vi "网络通信.vi"() -> ()   [LabVIEW 2015]
panel:
  in  "目标IP":string caption="连接对象"
  in  "端口":u16
  in  "UDP连接":refnum<k16>
  in  "连接对象":u16(ring) items=["no connection"]
  in  "Multi Client ID":T1
  out "状态显示":string
  out "发送数据":i32
  in  "连接协议":enum16{"TCP Client", "TCP Server", "UDP"}(ring)
  in  "清空接收":bool
  in  "端口号":u16=1 caption="端 口 号:"
  in  "IP地址":string caption="IP  地 址"
  in  "连接":bool
  in  "发送":bool
  in  "数据接收":string
  in  "数据发送":string
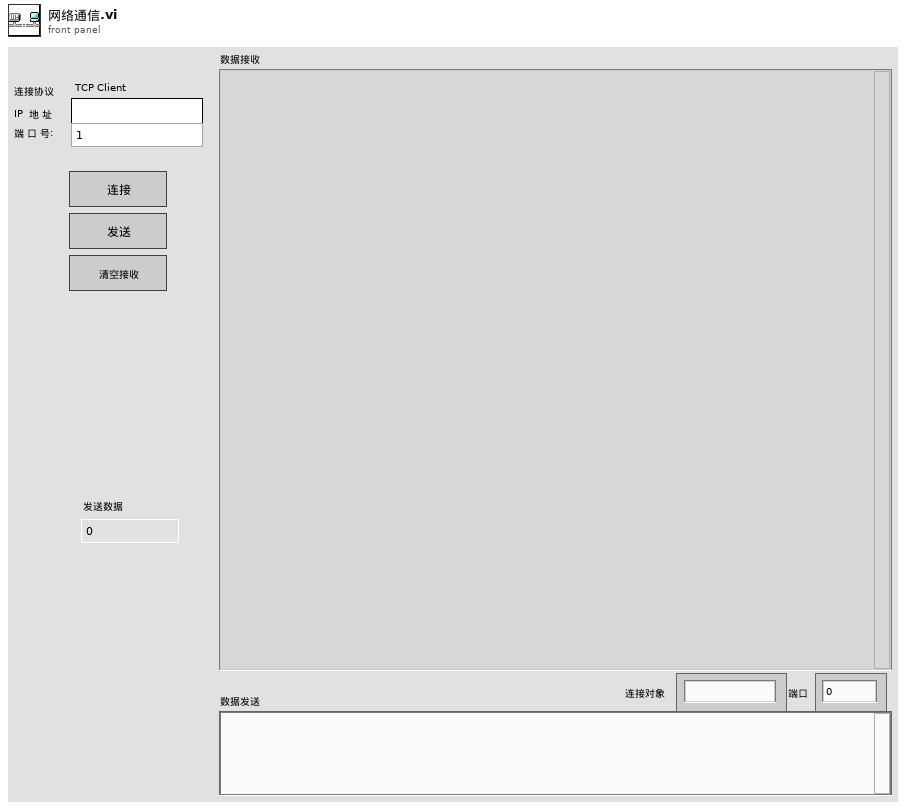
[diagram p1: front panel]
types:
  T1 = cluster{"Client":refnum<k5>[], "侦听器ID":refnum<k5>, "远程连接对象":cluster{"IP":string, "端口":u16}[]}
  T2 = enum16{"Initialization", "IDLE", "Connect", "S_Connect", "C_Read/Write", "C_Disconnect", "S_Read/Write", "S_Disconnect"}
  T3 = enum8{"Enabled", "Disabled", "Disabled and Grayed Out"}
  T4 = typedef "LVRectTypeDef.ctl" = cluster{"Left":i16, "Top":i16, "Right":i16, "Bottom":i16}
  T5 = typedef "LVPointTypeDef.ctl" = cluster{"Horizontal":i16, "Vertical":i16}
  T6 = cluster{"remote address":string, "remote port":u16}
  T7 = cluster{"remote address":string, "remote port":u16}[]
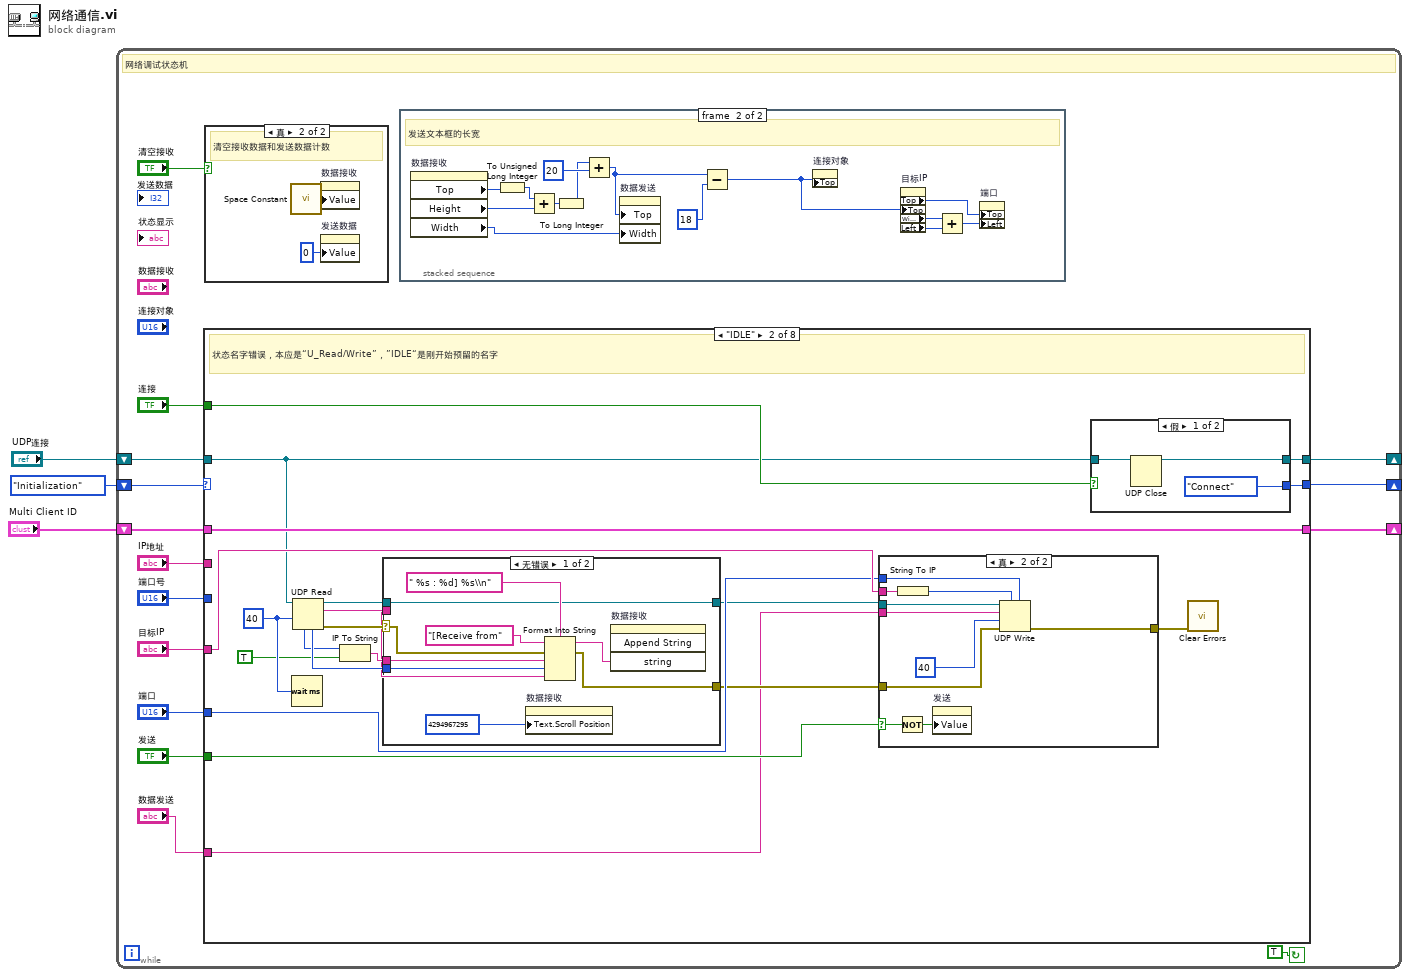
[diagram p0: block diagram]
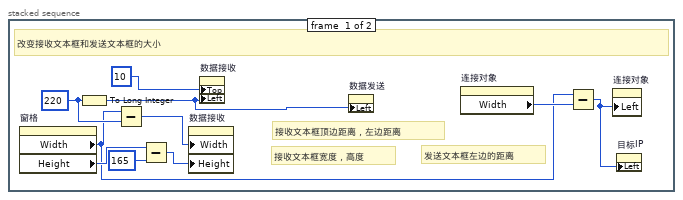
[diagram p2: hidden frame]
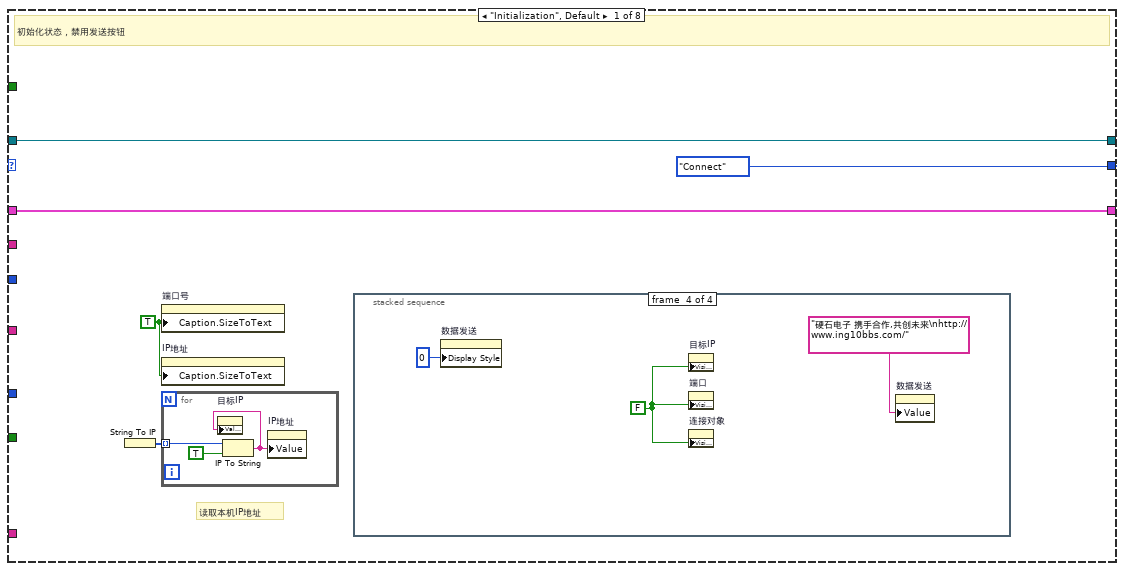
[diagram p4: hidden frame]
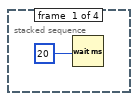
[diagram p5: hidden frame]
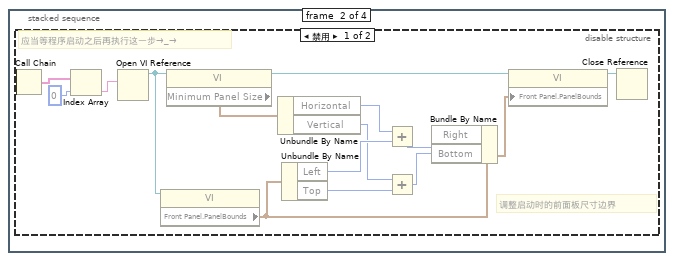
[diagram p6: hidden frame]
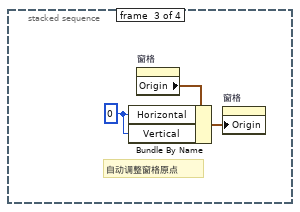
[diagram p8: hidden frame]
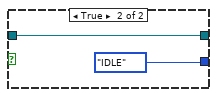
[diagram p9: hidden frame]
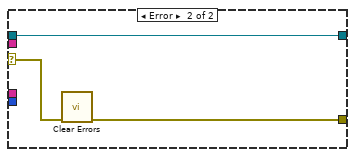
[diagram p11: hidden frame]
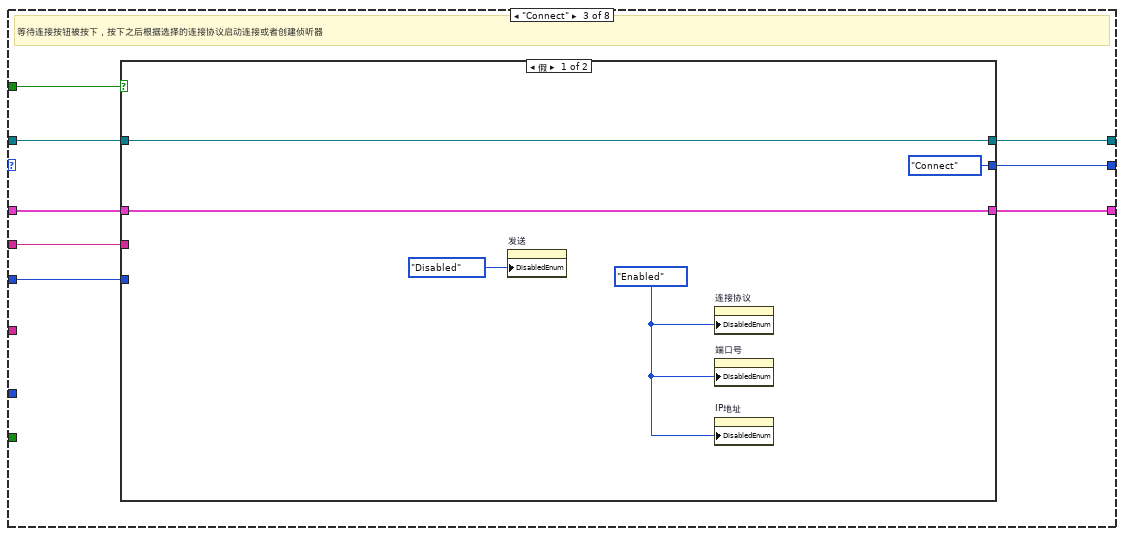
[diagram p12: hidden frame]
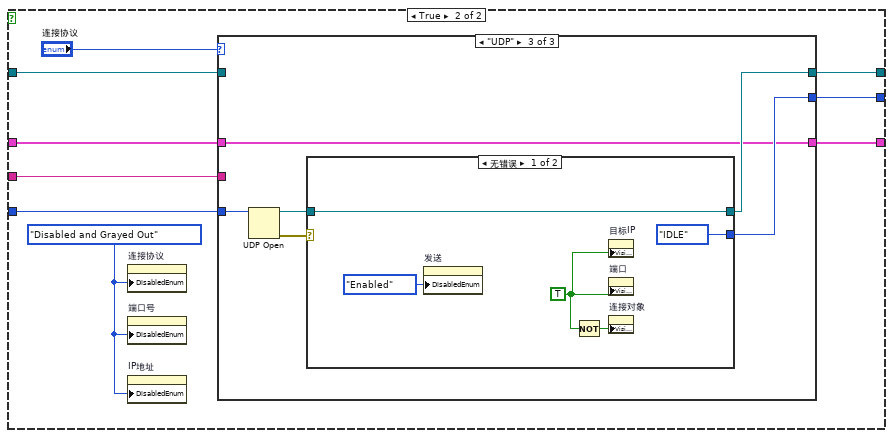
[diagram p13: hidden frame]
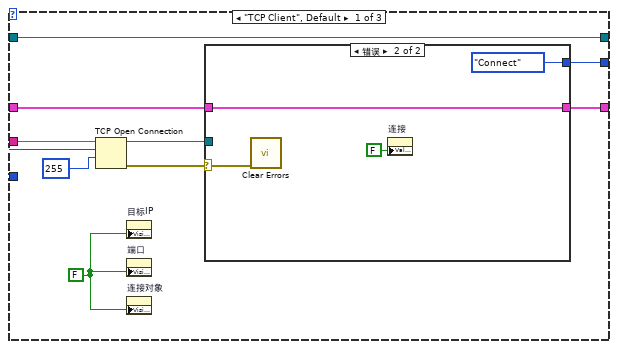
[diagram p14: hidden frame]
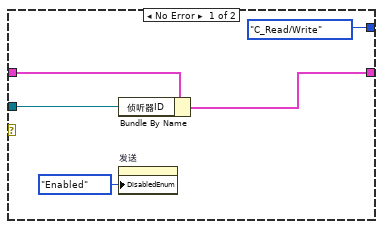
[diagram p15: hidden frame]
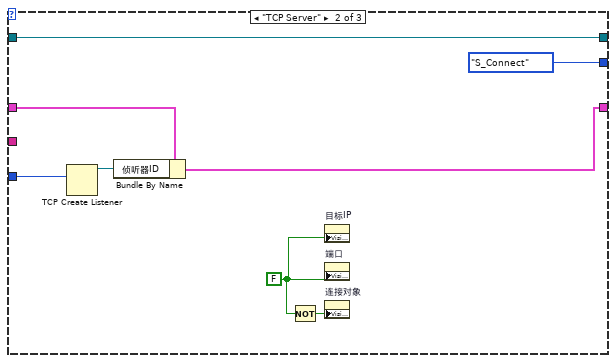
[diagram p16: hidden frame]
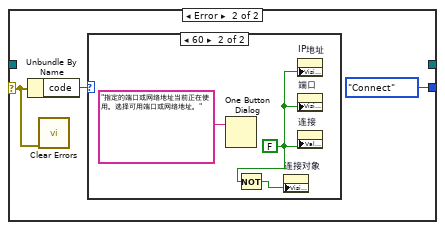
[diagram p17: hidden frame]
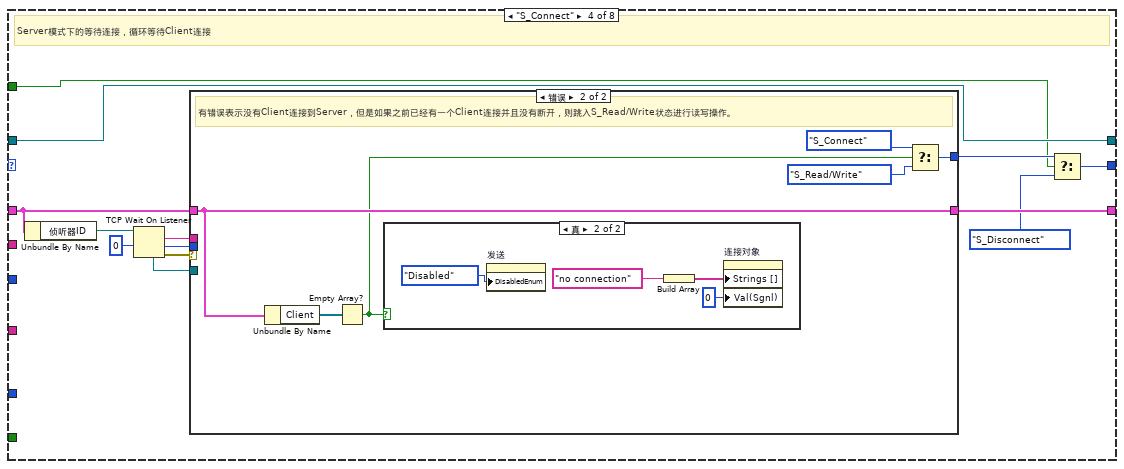
[diagram p19: hidden frame]
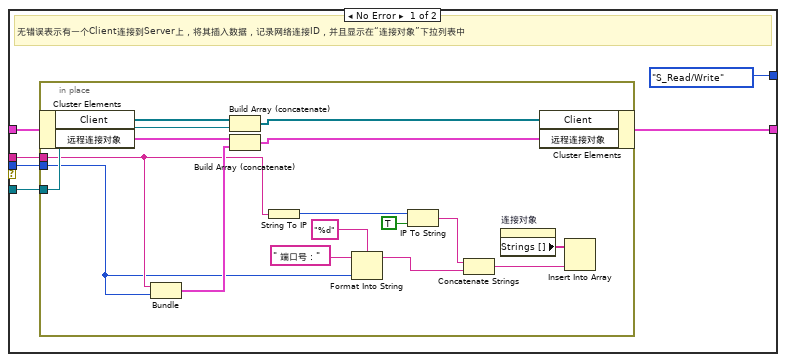
[diagram p20: hidden frame]
diagram:
  n1 = while "While循环" {
    shift-right: [w14] -> _
    shift-left: "Multi Client ID" -> [w15]
    shift-right: [w12] -> _
    shift-left: T2."Initialization" -> [w13]
    shift-right: [w9] -> _
    shift-left: "UDP连接" -> [w10]
    stop <- TRUE continue-if-true
    # "网络调试状态机"
    n2 = case "条件结构" shown="\"IDLE\"" w13 {
      tunnel: "IP地址" -> [_ _ w131 _ _ _ _ _]
      tunnel: "端口号" -> [_ _ w130 _ _ _ _ _]
      tunnel: w15 -> [w49 w94 w129 w198 w242 w267 w281 w344]
      tunnel: [w49 w94 w128 w197 w242 w267 w280 w344] -> w14
      tunnel: [T2."Connect" w93 w127 w192 w249 T2."Connect" w279 T2."Connect"] -> w12
      tunnel: w10 -> [w47 w76 w126 w191 w239 w266 w276 w338]
      tunnel: [w47 w75 w125 w191 w239 w266 w276 w338] -> w9
      tunnel: "目标IP" -> [_ w89 _ _ _ _ _ _]
      tunnel: "端口" -> [_ w88 _ _ _ _ _ _]
      tunnel: "发送" -> [_ w79 _ _ w238 _ w274 _]
      tunnel: "连接" -> [_ w77 w124 w190 w237 _ w273 _]
      tunnel: "数据发送" -> [_ w78 _ _ w236 _ w272 _]
      frame "Initialization", Default {
        w45 = TRUE
        # "读取本机IP地址"
        # "初始化状态，禁用发送按钮"
        n3 = String To IP() -> (0:w46:u32[])  [unwired: 1 out]
        n4 = property on="端口号" class="DigNum (严格)"("Caption.SizeToText"=w45) -> ()  [unwired: 2 in, 2 out]
        n5 = property on="IP地址" class="Str"("Caption.SizeToText"=w45) -> ()  [unwired: 2 in, 2 out]
        n6 = for {
          tunnel: w46 -> [w73] mode=indexing
          n7 = IP To String(1:TRUE ("dot notation? (F)"), 2:w73) -> (0:w72:string)
          n8 = property on="目标IP" class="Str"("Value"=w72) -> ()  [unwired: 2 in, 2 out]
          n9 = property on="IP地址" class="Str"("Value"=w72) -> ()  [unwired: 2 in, 2 out]
        }
        n10 = stacked-sequence {
          frame #0 {
            n11 = Wait (ms)(milliseconds to wait=u32 20) -> ()  [unwired: 1 out]
          }
          frame #1 {
            n12 = disable-structure shown="禁用" {
              frame Disabled {
                # "调整启动时的前面板尺寸边界"
                # "应当等程序启动之后再执行这一步→_→"
                n13 = Call Chain ("调用链")() -> (call chain=w53:string[])
                n14 = Index Array(array=w53, index=0) -> (element=w51:string)
                n15 = Open VI Reference(vi path=w51) -> (vi reference=w63:refnum<vi>)  [unwired: 1 in, 5 out]
                n16 = property class="VI"(reference=w63) -> ("Front Panel.PanelBounds"=w60:T4)  [unwired: 1 in, 2 out]
                n17 = property class="VI"(reference=w63) -> (reference out=w64:refnum<vi>, "Minimum Panel Size"=w54:T5)  [unwired: 1 in, 1 out]
                n18 = Unbundle By Name(w54) -> ("Horizontal"=w61:i16, "Vertical"=w58:i16)
                n19 = Unbundle By Name(w60) -> ("Left"=w62:i16, "Top"=w57:i16)
                n20 = Add(x=w61, y=w62) -> (x+y=w59:i16)
                n21 = Add(x=w58, y=w57) -> (x+y=w56:i16)
                n22 = Bundle By Name(cluster=w60, "Right"=w59, "Bottom"=w56) -> (w55:T4)
                n23 = property class="VI"(reference=w64, "Front Panel.PanelBounds"=w55) -> (reference out=w65:refnum<vi>)  [unwired: 1 in, 1 out]
                n24 = Close Reference(reference=w65) -> ()  [unwired: 1 in, 1 out]
              }
              frame Enabled {
              }
            }
          }
          frame #2 {
            w68 = i16 0
            # "自动调整窗格原点"
            n25 = property on="窗格" class="Pane"() -> ("Origin"=w67:T5)  [unwired: 2 in, 2 out]
            n26 = Bundle By Name(cluster=w67, "Horizontal"=w68, "Vertical"=w68) -> (w66:T5)
            n27 = property on="窗格" class="Pane"("Origin"=w66) -> ()  [unwired: 2 in, 2 out]
          }
          frame #3 {
            w69 = FALSE
            n28 = property on="数据发送" class="Str"("Display Style"=u32 0) -> ()  [unwired: 2 in, 2 out]
            n29 = property on="目标IP" class="Str"("Visible"=w69) -> ()  [unwired: 2 in, 2 out]
            n30 = property on="端口" class="DigNum (严格)"("Visible"=w69) -> ()  [unwired: 2 in, 2 out]
            n31 = property on="连接对象" class="Ring (严格)"("Visible"=w69) -> ()  [unwired: 2 in, 2 out]
            n32 = property on="数据发送" class="Str"("Value"="硬石电子 携手合作,共创未来\nhttp://www.ing10bbs.com/") -> ()  [unwired: 2 in, 2 out]
          }
        }
      }
      frame "IDLE" {
        w87 = 40
        # "状态名字错误，本应是“U_Read/Write”，”IDLE“是刚开始预留的名字"
        n33 = Wait (ms)(milliseconds to wait=w87) -> ()  [unwired: 1 out]
        n34 = UDP Read(connection ID=w76, timeout ms (25000)=w87) -> (data out=w91:string, error out=w92:errorcluster, 3:w86:refnum<k16>, 4:w90:u16, 6:w84:u32)  [unwired: 2 in]
        n35 = IP To String(1:TRUE, 2:w84) -> (0:w82:string)
        n36 = case shown="无错误" w92 {
          selector: w92 -> [w116 w123]
          tunnel: w91 -> [w118 _]
          tunnel: w90 -> [w119 _]
          tunnel: [w115 w122] -> w85
          tunnel: w86 -> [w115 w122]
          tunnel: w82 -> [w113 _]
          tunnel: [w112 w121] -> w81
          frame No Error {
            n37 = property on="数据接收" class="Str"("Text.Scroll Position"=u32 4294967295) -> ()  [unwired: 2 in, 2 out]
            n38 = Format Into String(format string=" %s : %d] %s\\n", initial string="[Receive from", error in=w116, w113, w119, w118) -> (resulting string=w117:string, error out=w112:errorcluster)
            n39 = invoke on="数据接收" class="Str" method="Append String"("string"=w117) -> ()  [unwired: 3 in, 4 out]
          }
          frame Error {
            n40 = call <vilib>:"Clear Errors.vi"("error in (no error)"=w123) -> ("error out"=w121:errorcluster)  [unwired: 5 in, 1 out]
          }
        }
        n41 = case shown="真" w79 {
          selector: w79 -> [_ w105]
          tunnel: w89 -> [_ w110]
          tunnel: w88 -> [_ w108]
          tunnel: w85 -> [_ w107]
          tunnel: w81 -> [w100 w103]
          tunnel: [w100 w102] -> w80
          tunnel: w78 -> [_ w101]
          frame False {
          }
          frame True {
            n42 = Not(x=w105) -> (.not. x?=w104:bool)
            n43 = String To IP(1:w110) -> (0:w109:u32)
            n44 = property on="发送" class="Bool (严格)"("Value"=w104) -> ()  [unwired: 2 in, 2 out]
            n45 = UDP Write(address=w109, port or service name=w108, connection ID=w107, data in=w101, 8:w103, 9:40) -> (error out=w102:errorcluster)  [unwired: 1 out]
          }
        }
        n46 = case shown="假" w77 {
          tunnel: [T2."Connect" T2."IDLE"] -> w93
          tunnel: w76 -> [w96 w98]
          tunnel: [w95 w98] -> w75
          frame False {
            n47 = UDP Close(connection ID=w96) -> (connection ID out=w95:refnum<k16>)  [unwired: 1 in, 1 out]
          }
          frame True {
          }
        }
        n48 = call <vilib>:"Clear Errors.vi"("error in (no error)"=w80) -> ()  [unwired: 5 in, 2 out]
      }
      frame "Connect" {
        # "等待连接按钮被按下，按下之后根据选择的连接协议启动连接或者创建侦听器"
        n49 = case shown="假" w124 {
          tunnel: w131 -> [_ w144]
          tunnel: w130 -> [_ w143]
          tunnel: w129 -> [w136 w142]
          tunnel: [w136 w141] -> w128
          tunnel: [T2."Connect" w140] -> w127
          tunnel: w126 -> [w133 w139]
          tunnel: [w133 w138] -> w125
          frame False {
            w132 = T3."Enabled"
            n50 = property on="发送" class="Bool (严格)"("DisabledEnum"=T3."Disabled") -> ()  [unwired: 2 in, 2 out]
            n51 = property on="连接协议" class="Enum (严格)"("DisabledEnum"=w132) -> ()  [unwired: 2 in, 2 out]
            n52 = property on="端口号" class="DigNum (严格)"("DisabledEnum"=w132) -> ()  [unwired: 2 in, 2 out]
            n53 = property on="IP地址" class="Str"("DisabledEnum"=w132) -> ()  [unwired: 2 in, 2 out]
          }
          frame True {
            w137 = T3."Disabled and Grayed Out"
            n54 = property on="连接协议" class="Enum (严格)"("DisabledEnum"=w137) -> ()  [unwired: 2 in, 2 out]
            n55 = property on="端口号" class="DigNum (严格)"("DisabledEnum"=w137) -> ()  [unwired: 2 in, 2 out]
            n56 = property on="IP地址" class="Str"("DisabledEnum"=w137) -> ()  [unwired: 2 in, 2 out]
            n57 = case shown="\"UDP\"" "连接协议" {
              tunnel: w144 -> [w155 _ _]
              tunnel: w143 -> [w154 w172 w178]
              tunnel: w142 -> [w151 w171 w173]
              tunnel: [w149 w169 w173] -> w141
              tunnel: [w148 T2."S_Connect" w176] -> w140
              tunnel: w139 -> [w147 w167 _]
              tunnel: [w147 w167 w174] -> w138
              frame "TCP Client", Default {
                w146 = FALSE
                n58 = TCP Open Connection(address=w155, remote port or service name=w154, timeout ms (60000)=255) -> (connection ID=w150:refnum<k5>, error out=w152:errorcluster)  [unwired: 2 in]
                n59 = property on="目标IP" class="Str"("Visible"=w146) -> ()  [unwired: 2 in, 2 out]
                n60 = property on="端口" class="DigNum (严格)"("Visible"=w146) -> ()  [unwired: 2 in, 2 out]
                n61 = property on="连接对象" class="Ring (严格)"("Visible"=w146) -> ()  [unwired: 2 in, 2 out]
                n62 = case shown="错误" w152 {
                  selector: w152 -> [_ w164]
                  tunnel: [w158 w163] -> w149
                  tunnel: [T2."C_Read/Write" T2."Connect"] -> w148
                  tunnel: w151 -> [w160 w163]
                  tunnel: w150 -> [w159 _]
                  frame No Error {
                    n63 = Bundle By Name(cluster=w160, "侦听器ID"=w159) -> (w158:T1)
                    n64 = property on="发送" class="Bool (严格)"("DisabledEnum"=T3."Enabled") -> ()  [unwired: 2 in, 2 out]
                  }
                  frame Error {
                    n65 = call <vilib>:"Clear Errors.vi"("error in (no error)"=w164) -> ()  [unwired: 5 in, 2 out]
                    n66 = property on="连接" class="Bool (严格)"("Value"=FALSE) -> ()  [unwired: 2 in, 2 out]
                  }
                }
              }
              frame "TCP Server" {
                w166 = FALSE
                n67 = TCP Create Listener(10:w172) -> (3:w170:refnum<k5>)  [unwired: 4 in, 2 out]
                n68 = Bundle By Name(cluster=w171, "侦听器ID"=w170) -> (w169:T1)
                n69 = Not(x=w166) -> (.not. x?=w165:bool)
                n70 = property on="目标IP" class="Str"("Visible"=w166) -> ()  [unwired: 2 in, 2 out]
                n71 = property on="端口" class="DigNum (严格)"("Visible"=w166) -> ()  [unwired: 2 in, 2 out]
                n72 = property on="连接对象" class="Ring (严格)"("Visible"=w165) -> ()  [unwired: 2 in, 2 out]
              }
              frame "UDP" {
                n73 = UDP Open(11:w178) -> (port=w175:refnum<k16>, 0:w177:errorcluster)  [unwired: 4 in, 1 out]
                n74 = case shown="无错误" w177 {
                  selector: w177 -> [_ w184]
                  tunnel: [T2."IDLE" T2."Connect"] -> w176
                  tunnel: w175 -> [w182 _]
                  tunnel: [w182 _] -> w174
                  frame No Error {
                    w180 = TRUE
                    n75 = property on="发送" class="Bool (严格)"("DisabledEnum"=T3."Enabled") -> ()  [unwired: 2 in, 2 out]
                    n76 = Not(x=w180) -> (.not. x?=w179:bool)
                    n77 = property on="目标IP" class="Str"("Visible"=w180) -> ()  [unwired: 2 in, 2 out]
                    n78 = property on="端口" class="DigNum (严格)"("Visible"=w180) -> ()  [unwired: 2 in, 2 out]
                    n79 = property on="连接对象" class="Ring (严格)"("Visible"=w179) -> ()  [unwired: 2 in, 2 out]
                  }
                  frame Error {
                    n80 = Unbundle By Name(w184) -> ("code"=w185:i32)
                    n81 = call <vilib>:"Clear Errors.vi"("error in (no error)"=w184) -> ()  [unwired: 5 in, 2 out]
                    n82 = case shown="60" w185 {
                      frame 0, Default {
                      }
                      frame 60 {
                        w187 = FALSE
                        n83 = One Button Dialog(message="指定的端口或网络地址当前正在使用。选择可用端口或网络地址。") -> ()  [unwired: 1 in, 1 out]
                        n84 = Not(x=w187) -> (.not. x?=w188:bool)
                        n85 = property on="连接对象" class="Ring (严格)"("Visible"=w188) -> ()  [unwired: 2 in, 2 out]
                        n86 = property on="IP地址" class="Str"("Visible"=w187) -> ()  [unwired: 2 in, 2 out]
                        n87 = property on="端口" class="DigNum (严格)"("Visible"=w187) -> ()  [unwired: 2 in, 2 out]
                        n88 = property on="连接" class="Bool (严格)"("Value"=w187) -> ()  [unwired: 2 in, 2 out]
                      }
                    }
                  }
                }
              }
            }
          }
        }
      }
      frame "S_Connect" {
        # "Server模式下的等待连接，循环等待Client连接"
        n89 = Unbundle By Name(w198) -> ("侦听器ID"=w201:refnum<k5>)
        n90 = TCP Wait On Listener(9:0 ("超时时间(ms)"), 11:w201) -> (0:w202:errorcluster, 1:w196:u16, 2:w195:string, 4:w199:refnum<k5>)  [unwired: 2 in, 1 out]
        n91 = case "条件结构" shown="错误" w202 {
          tunnel: w199 -> [w208 _]
          tunnel: w198 -> [w204 w228]
          tunnel: [w206 w228] -> w197
          tunnel: [T2."S_Read/Write" w229] -> w193
          tunnel: w196 -> [w205 _]
          tunnel: w195 -> [w203 _]
          frame No Error {
            # "无错误表示有一个Client连接到Server上，将其插入数据，记录网络连接ID，并且显示在“连接对象”下拉列表中"
            n92 = in-place {
              in-place-border: w208 -> [w222]
              in-place-border: w205 -> [w211]
              in-place-border: w203 -> [w212]
              n93 = in-place-cluster #1(w204) -> ("Client"=w224:refnum<k5>[], "远程连接对象"=w215:cluster{"IP":string, "端口":u16}[])
              n94 = Bundle("remote address"=w212, "remote port"=w211) -> (w213:T6)  [unwired: 1 in]
              n95 = Build Array (concatenate)(w224, w222) -> (w223:refnum<k5>[])
              n96 = Build Array (concatenate)(w215, w213) -> (w214:T7)
              n97 = String To IP(1:w212) -> (0:w216:u32)
              n98 = Format Into String(format string="%d", initial string=" 端口号：", w211) -> (resulting string=w221:string)  [unwired: 1 in, 1 out]
              n99 = IP To String(1:TRUE, 2:w216) -> (0:w218:string)
              n100 = Concatenate Strings(w218, w221) -> (w210:string)
              n101 = property on="连接对象" class="Ring (严格)"() -> ("Strings []"=w209:string[])  [unwired: 2 in, 2 out]
              n102 = in-place-cluster #1("Client"=w223, "远程连接对象"=w214) -> (w206:T1)
              n103 = Insert Into Array(array=w209, new element=w210) -> ()  [unwired: 1 in, 1 out]
            }
          }
          frame Error {
            # "有错误表示没有Client连接到Server，但是如果之前已经有一个Client连接并且没有断开，则跳入S_Read/Write状态进行读写操作。"
            n104 = Unbundle By Name(w228) -> ("Client"=w230:refnum<k5>[])
            n105 = Empty Array?(array=w230) -> (empty?=w225:bool)
            n106 = case shown="真" w225 {
              frame False {
                n107 = property on="发送" class="Bool (严格)"("DisabledEnum"=T3."Enabled") -> ()  [unwired: 2 in, 2 out]
              }
              frame True {
                n108 = property on="发送" class="Bool (严格)"("DisabledEnum"=T3."Disabled") -> ()  [unwired: 2 in, 2 out]
                n109 = Build Array("no connection") -> (w234:string[])
                n110 = property on="连接对象" class="Ring (严格)"("Strings []"=w234, "Val(Sgnl)"=u16 0) -> ()  [unwired: 2 in, 2 out]
              }
            }
            n111 = Select(t=T2."S_Connect", s=w225, f=T2."S_Read/Write") -> (s? t:f=w229:T2)
          }
        }
        n112 = Select(t=w193, s=w190, f=T2."S_Disconnect") -> (s? t:f=w192:T2)
      }
      frame "C_Read/Write" {
        # "Client 模式下的读写状态"
        n113 = Unbundle By Name(w242) -> ("侦听器ID"=w243:refnum<k5>)
        n114 = TCP Read(connection ID=w243, bytes to read=1, 9:0) -> (connection ID out=w245:refnum<k5>, data out=w246:string, error out=w247:errorcluster)  [unwired: 2 in]
        n115 = case shown="无错误" w247 {
          selector: w247 -> [_ w260]
          tunnel: w246 -> [w259 _]
          tunnel: w245 -> [_ w261]
          frame No Error {
            # "无错误，能读取到数据"
            n116 = invoke on="数据接收" class="Str" method="Append String"("string"=w259) -> ()  [unwired: 3 in, 4 out]
            n117 = property on="数据接收" class="Str"("Text.Scroll Position"=u32 4294967295) -> ()  [unwired: 2 in, 2 out]
          }
          frame Error {
            # "有错误，但超时可以忽略"
            n118 = Unbundle By Name(w260) -> ("code"=w262:i32)
            n119 = case shown="66" w262 {
              tunnel: w261 -> [_ _ _]
              tunnel: w260 -> [w263 _ w265]
              frame 0, Default {
                # "其他错误"
                n120 = call <vilib>:"Clear Errors.vi"("error in (no error)"=w263) -> ()  [unwired: 5 in, 2 out]
              }
              frame 56 {
                # "连接超时，表示无错误"
              }
              frame 66 {
                # "断开连接"
                n121 = call <vilib>:"Clear Errors.vi"("error in (no error)"=w265) -> ()  [unwired: 5 in, 2 out]
                n122 = property on="连接" class="Bool (严格)"("Value"=FALSE) -> ()  [unwired: 2 in, 2 out]
              }
            }
          }
        }
        n123 = case shown="真" w238 {
          selector: w238 -> [_ w255]
          tunnel: w243 -> [_ w257]
          tunnel: w236 -> [_ w250]
          frame False {
          }
          frame True {
            n124 = Not(x=w255) -> (.not. x?=w254:bool)
            n125 = property on="发送" class="Bool (严格)"("Value"=w254) -> ()  [unwired: 2 in, 2 out]
            n126 = TCP Write(connection ID=w257, data in=w250) -> (bytes written=w252:i32, error out=w256:errorcluster)  [unwired: 2 in, 1 out]
            n127 = call <vilib>:"Clear Errors.vi"("error in (no error)"=w256) -> ()  [unwired: 5 in, 2 out]
            n128 = property on="发送数据" class="DigNum (严格)"() -> ("Value"=w253:i32)  [unwired: 2 in, 2 out]
            n129 = Add(x=w253, y=w252) -> (x+y=w251:i32)
            n130 = property on="发送数据" class="DigNum (严格)"("Value"=w251) -> ()  [unwired: 2 in, 2 out]
          }
        }
        n131 = Select(t=T2."C_Read/Write", s=w237, f=T2."C_Disconnect") -> (s? t:f=w249:T2)
      }
      frame "C_Disconnect" {
        # "Client 模式下的断开连接状态，进入这个状态只有两种可能，一种是Server 断开连接，另一种是Client主动断开连接（按下断开连接按钮）"
        n132 = Unbundle By Name(w267) -> ("侦听器ID"=w271:refnum<k5>)
        n133 = TCP Close Connection(connection ID=w271) -> (error out=w270:errorcluster)  [unwired: 2 in, 1 out]
        n134 = call <vilib>:"Clear Errors.vi"("error in (no error)"=w270) -> ()  [unwired: 5 in, 2 out]
        n135 = property on="发送" class="Bool (严格)"("DisabledEnum"=T3."Disabled") -> ()  [unwired: 2 in, 2 out]
      }
      frame "S_Read/Write" {
        # "状态机实现Server模式的读写状态，轮询各个Client的数据，有数据则显示，无数据则超时无响应，如果断开连接则删除网络连接句柄ID。写数据到Client的时候，则根据下拉列表所选择的Client作为连接对象。"
        n136 = in-place {
          in-place-border: [w292] -> w275
          n137 = in-place-cluster #2(w281) -> ("Client"=w292:refnum<k5>[], "远程连接对象"=w294:cluster{"IP":string, "端口":u16}[])
          n138 = for {
            tunnel: [w311] -> w296 mode=indexing if=w299
            tunnel: w292 -> [w310] mode=indexing
            tunnel: w294 -> [w298] mode=indexing
            tunnel: [w308] -> w295 mode=indexing if=w299
            tunnel: [w297] -> w293 mode=indexing if=w299
            n139 = TCP Read(connection ID=w310, bytes to read=1, 9:0) -> (connection ID out=w312:refnum<k5>, data out=w313:string, error out=w314:errorcluster)  [unwired: 2 in]
            n140 = case "条件结构" shown="无错误" w314 {
              selector: w314 -> [_ w324]
              tunnel: w313 -> [w320 _]
              tunnel: w312 -> [w319 w326]
              tunnel: [w319 w325] -> w311
              tunnel: [TRUE w323] -> w299
              tunnel: [w318 w322] -> w308
              tunnel: w298 -> [w318 w321]
              frame No Error {
                # "无错误，能读取到数据"
                # "Client有发送数据，追加到接受文本框字符串结尾"
                n141 = invoke on="数据接收" class="Str" method="Append String"("string"=w320) -> ()  [unwired: 3 in, 4 out]
                n142 = property on="数据接收" class="Str"("Text.Scroll Position"=u32 4294967295) -> ()  [unwired: 2 in, 2 out]
              }
              frame Error {
                # "有错误，但超时可以忽略"
                n143 = Unbundle By Name(w324) -> ("code"=w327:i32)
                n144 = case "条件结构" shown="66" w327 {
                  tunnel: w326 -> [_ w332 w337]
                  tunnel: [_ w332 _] -> w325
                  tunnel: w324 -> [w329 _ w334]
                  tunnel: [FALSE TRUE FALSE] -> w323
                  tunnel: [_ w331 _] -> w322
                  tunnel: w321 -> [_ w331 _]
                  frame 0, Default {
                    # "其他错误"
                    n145 = call <vilib>:"Clear Errors.vi"("error in (no error)"=w329) -> ()  [unwired: 5 in, 2 out]
                  }
                  frame 56 {
                    # "连接超时，表示无错误"
                    # "超时错误，当没有断开连接，只是Client没有发送数据而已"
                  }
                  frame 66 {
                    # "断开连接"
                    # "Client 断开连接，关闭连接，注销句柄ID"
                    n146 = TCP Close Connection(connection ID=w337, error in (no error)=w334) -> (error out=w333:errorcluster)  [unwired: 1 in, 1 out]
                    n147 = call <vilib>:"Clear Errors.vi"("error in (no error)"=w333) -> ()  [unwired: 5 in, 2 out]
                    n148 = property on="连接对象" class="Ring (严格)"("Val(Sgnl)"=0) -> ()  [unwired: 2 in, 2 out]
                  }
                }
              }
            }
            n149 = Unbundle(w308) -> ("IP"=w307:string, "端口"=w300:u16)
            n150 = String To IP(1:w307) -> (0:w306:u32)
            n151 = Format Into String(format string="%d", initial string=" 端口号：", w300) -> (resulting string=w304:string)  [unwired: 1 in, 1 out]
            n152 = IP To String(1:TRUE, 2:w306) -> (0:w301:string)
            n153 = Concatenate Strings(w301, w304) -> (w297:string)
          }
          n154 = in-place-cluster #2("Client"=w296, "远程连接对象"=w295) -> (w280:T1)
          n155 = property on="连接对象" class="Ring (严格)"("Strings []"=w293) -> ()  [unwired: 2 in, 2 out]
        }
        n156 = case "条件结构" shown="真" w274 {
          selector: w274 -> [_ w290]
          tunnel: w275 -> [_ w289]
          tunnel: w272 -> [_ w282]
          frame False {
          }
          frame True {
            # "发送数据，根据下拉列表的内容来选择发送数据的对象"
            n157 = property on="连接对象" class="Ring (严格)"() -> ("Value"=w286:u16)  [unwired: 2 in, 2 out]
            n158 = Not(x=w290) -> (.not. x?=w291:bool)
            n159 = property on="发送" class="Bool (严格)"("Value"=w291) -> ()  [unwired: 2 in, 2 out]
            n160 = Index Array(array=w289, index=w286) -> (element=w288:refnum<k5>)
            n161 = TCP Write(connection ID=w288, data in=w282) -> (bytes written=w284:i32, error out=w287:errorcluster)  [unwired: 2 in, 1 out]
            n162 = property on="发送数据" class="DigNum (严格)"() -> ("Value"=w285:i32)  [unwired: 2 in, 2 out]
            n163 = call <vilib>:"Clear Errors.vi"("error in (no error)"=w287) -> ()  [unwired: 5 in, 2 out]
            n164 = Add(x=w285, y=w284) -> (x+y=w283:i32)
            n165 = property on="发送数据" class="DigNum (严格)"("Value"=w283) -> ()  [unwired: 2 in, 2 out]
          }
        }
        n166 = Select(t=T2."S_Connect", s=w273, f=T2."S_Disconnect") -> (s? t:f=w279:T2)
      }
      frame "S_Disconnect" {
        w340 = u16 0
        # "Server状态下断开连接，关闭所有连接句柄，注销网络连接ID"
        n167 = Unbundle By Name(w344) -> ("Client"=w348:refnum<k5>[], "侦听器ID"=w349:refnum<k5>)
        n168 = TCP Close Connection(connection ID=w349) -> (error out=w347:errorcluster)  [unwired: 2 in, 1 out]
        n169 = for {
          tunnel: w348 -> [w352] mode=indexing
          shift-right: [w350] -> w346
          shift-left: w347 -> [w351]
          n170 = TCP Close Connection(connection ID=w352, error in (no error)=w351) -> (error out=w350:errorcluster)  [unwired: 1 in, 1 out]
        }
        n171 = property on="发送" class="Bool (严格)"("DisabledEnum"=T3."Disabled") -> ()  [unwired: 2 in, 2 out]
        n172 = property on="连接对象" class="Ring (严格)"("Val(Sgnl)"=w340) -> ()  [unwired: 2 in, 2 out]
        n173 = Bundle("no connection", w340) -> (w342:cluster{string, u16})  [unwired: 1 in]
        n174 = call <vilib>:"Clear Errors.vi"("error in (no error)"=w346) -> ()  [unwired: 5 in, 2 out]
        n175 = Build Array(w342) -> (w341:cluster{string, u16}[])
        n176 = property on="连接对象" class="Ring (严格)"("StringsAndValues[]"=w341) -> ()  [unwired: 2 in, 2 out]
      }
    }
    n177 = case "条件结构" shown="真" "清空接收" {
      frame False {
      }
      frame True {
        # "清空接收数据和发送数据计数"
        n178 = call <vilib>:"Space Constant.vi"() -> ("String"=w44:string)
        n179 = property on="数据接收" class="Str"("Value"=w44) -> ()  [unwired: 2 in, 2 out]
        n180 = property on="发送数据" class="DigNum (严格)"("Value"=0) -> ()  [unwired: 2 in, 2 out]
      }
    }
    n181 = stacked-sequence "层叠式顺序结构" {
      frame #0 {
        w24 = u32 220
        # "接收文本框顶边距离，左边距离"
        # "接收文本框宽度，高度"
        # "发送文本框左边的距离"
        # "改变接收文本框和发送文本框的大小"
        n182 = property on="窗格" class="Pane"() -> ("Width"=w20:u32, "Height"=w28:u32)  [unwired: 2 in, 2 out]
        n183 = To Long Integer(number=w24) -> (32bit integer=w22:i32)
        n184 = Subtract(x=w20, y=w24) -> (x-y=w26:u32)
        n185 = Subtract(x=w28, y=u32 165) -> (x-y=w27:u32)
        n186 = property on="数据接收" class="Str"("Width"=w26, "Height"=w27) -> ()  [unwired: 2 in, 2 out]
        n187 = property on="数据接收" class="Str"("Top"=10, "Left"=w22) -> ()  [unwired: 2 in, 2 out]
        n188 = property on="数据发送" class="Str"("Left"=w22) -> ()  [unwired: 2 in, 2 out]
        n189 = property on="连接对象" class="Ring (严格)"() -> ("Width"=w21:u32)  [unwired: 2 in, 2 out]
        n190 = Subtract(x=w20, y=w21) -> (x-y=w19:u32)
        n191 = property on="连接对象" class="Ring (严格)"("Left"=w19) -> ()  [unwired: 2 in, 2 out]
        n192 = property on="目标IP" class="Str"("Left"=w19) -> ()  [unwired: 2 in, 2 out]
      }
      frame #1 {
        # "发送文本框的长宽"
        n193 = property on="数据接收" class="Str"() -> ("Top"=w41:i32, "Height"=w42:u32, "Width"=w37:u32)  [unwired: 2 in, 2 out]
        n194 = To Unsigned Long Integer(number=w41) -> (unsigned 32bit integer=w40:u32)
        n195 = Add(x=w40, y=w42) -> (x+y=w39:u32)
        n196 = To Long Integer(number=w39) -> (32bit integer=w34:i32)
        n197 = Add(x=w34, y=20) -> (x+y=w36:i32)
        n198 = property on="数据发送" class="Str"("Top"=w36, "Width"=w37) -> ()  [unwired: 2 in, 2 out]
        n199 = Subtract(x=w36, y=18) -> (x-y=w30:i32)
        n200 = property on="连接对象" class="Ring (严格)"("Top"=w30) -> ()  [unwired: 2 in, 2 out]
        n201 = property on="目标IP" class="Str"("Top"=w30) -> ("Top"=w29:i32, "Width"=w33:u32, "Left"=w32:i32)  [unwired: 2 in, 2 out]
        n202 = Add(x=w33, y=w32) -> (x+y=w31:u32)
        n203 = property on="端口" class="DigNum (严格)"("Top"=w29, "Left"=w31) -> ()  [unwired: 2 in, 2 out]
      }
    }
  }
